vi "Match String.vi"(8 "Offset (0)":i32, 9 "Pattern":string, 11 "Source":string) -> (2 "Match?":bool, 3 "String Match":T1)   [LabVIEW 2016, in "Suggestion Box.lvclass"]
doc: "Searches in <b>Source</b> for <b>Pattern</b> starting at <b>Offset</b>.\n--------------------\nCopyright (c) 2019 Analog Devices, Inc. All rights reserved.\n\nRedistribution and use in source and binary forms, with or without modification,\nare permitted provided that the following conditions are met:\n - Redistributions of source code must retain the above copyright notice, this\n list of conditions and the following disclaimer.\n - Redistributions in binary form must reproduce the above copyright notice,\n this list of conditions and the following disclaimer in the documentation\n and/or other materials provided with the distribution.\n - Modified versions of the software must be conspicuously marked as such.\n - This software is licensed solely and exclusively for use with\n processors/products manufactured by or for Analog Devices, Inc.\n - This software may not be combined or merged with other code in any manner\n that would cause the software to become subject to terms and conditions\n which differ from those listed here.\n - Neither the name of Analog Devices, Inc. nor the names of its contributors\n may be used to endorse or promote products derived from this software\n without specific prior written permission.\n - The use of this software may or may not infringe the patent rights of one or\n more patent holders. This license does not release you from the requirement\n that you obtain separate licenses from these patent holders to use this\n software.\n\nTHIS SOFTWARE IS PROVIDED BY ANALOG DEVICES, INC. AND CONTRIBUTORS \"AS IS\" AND\nANY EXPRESS OR IMPLIED WARRANTIES, INCLUDING, BUT NOT LIMITED TO,\nNON-INFRINGEMENT, TITLE, MERCHANTABILITY AND FITNESS FOR A PARTICULAR PURPOSE\nARE DISCLAIMED. IN NO EVENT SHALL ANALOG DEVICES, INC. OR CONTRIBUTORS BE LIABLE\nFOR ANY DIRECT, INDIRECT, INCIDENTAL, SPECIAL, EXEMPLARY, PUNITIVE OR\nCONSEQUENTIAL DAMAGES (INCLUDING, BUT NOT LIMITED TO, DAMAGES ARISING OUT OF\nCLAIMS OF INTELLECTUAL PROPERTY RIGHTS INFRINGEMENT; PROCUREMENT OF SUBSTITUTE\nGOODS OR SERVICES; LOSS OF USE, DATA, OR PROFITS; OR BUSINESS INTERRUPTION)\nHOWEVER CAUSED AND ON ANY THEORY OF LIABILITY, WHETHER IN CONTRACT, STRICT\nLIABILITY, OR TORT (INCLUDING NEGLIGENCE OR OTHERWISE) ARISING IN ANY WAY OUT OF\nTHE USE OF THIS SOFTWARE, EVEN IF ADVISED OF THE POSSIBILITY OF SUCH DAMAGE.\n\n2019-01-10-7CBSD SLA"
uses:
  Suggestion Box.lvclass
  String Match.ctl
  Segment.ctl
panel:
  # "Copyright (c) 2019 Analog Devices, Inc.  All rights reserved.\n\nRedistribution and use in source and binary forms, with or without modification,\nare permitted provided that the following conditions are met:\n  - Redistributions of source code must retain the above copyright notice, this\n    list of conditions and the following disclaimer.\n  - Redistributions in binary form must reproduce the above copyright notice,\n    this list of conditions and the following disclaimer in the documentation\n    and/or other materials provided with the distribution.\n  - Modified versions of the software must be conspicuously marked as such.\n  - This software is licensed solely and exclusively for use with\n    processors/products manufactured by or for Analog Devices, Inc.\n  - This software may not be combined or merged with other code in any manner\n    that would cause the software to become subject to terms and conditions\n    which differ from those listed here.\n  - Neither the name of Analog Devices, Inc. nor the names of its contributors\n    may be used to endorse or promote products derived from this software\n    without specific prior written permission.\n  - The use of this software may or may not infringe the patent rights of one or\n    more patent holders.  This license does not release you from the requirement\n    that you obtain separate licenses from these patent holders to use this\n    software.\n\nTHIS SOFTWARE IS PROVIDED BY ANALOG DEVICES, INC. AND CONTRIBUTORS \"AS IS\" AND\nANY EXPRESS OR IMPLIED WARRANTIES, INCLUDING, BUT NOT LIMITED TO,\nNON-INFRINGEMENT, TITLE, MERCHANTABILITY AND FITNESS FOR A PARTICULAR PURPOSE\nARE DISCLAIMED. IN NO EVENT SHALL ANALOG DEVICES, INC. OR CONTRIBUTORS BE LIABLE\nFOR ANY DIRECT, INDIRECT, INCIDENTAL, SPECIAL, EXEMPLARY, PUNITIVE OR\nCONSEQUENTIAL DAMAGES (INCLUDING, BUT NOT LIMITED TO, DAMAGES ARISING OUT OF\nCLAIMS OF INTELLECTUAL PROPERTY RIGHTS INFRINGEMENT; PROCUREMENT OF SUBSTITUTE\nGOODS OR SERVICES; LOSS OF USE, DATA, OR PROFITS; OR BUSINESS INTERRUPTION)\nHOWEVER CAUSED AND ON ANY THEORY OF LIABILITY, WHETHER IN CONTRACT, STRICT\nLIABILITY, OR TORT (INCLUDING NEGLIGENCE OR OTHERWISE) ARISING IN ANY WAY OUT OF\nTHE USE OF THIS SOFTWARE, EVEN IF ADVISED OF THE POSSIBILITY OF SUCH DAMAGE.\n\n2019-01-10-7CBSD SLA"
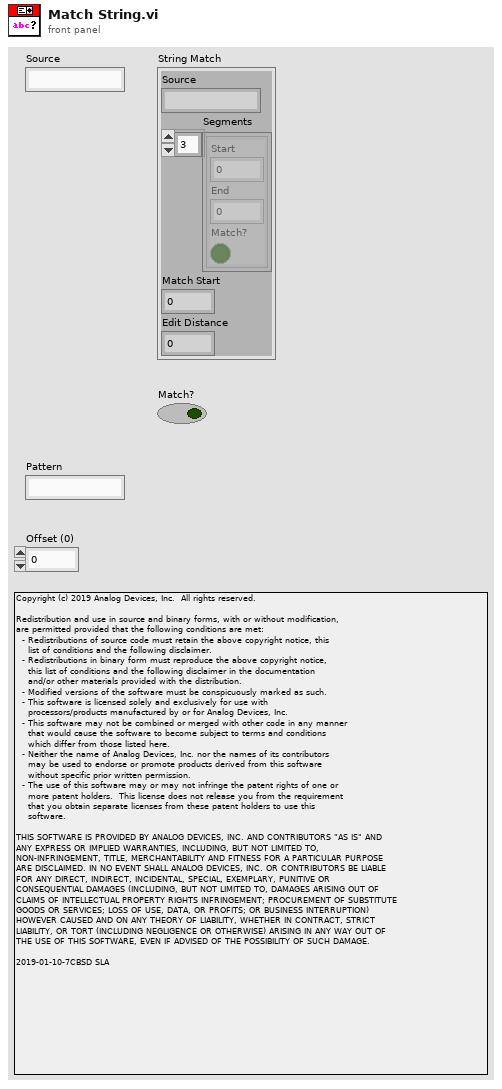
[diagram p1: front panel]
types:
  T1 = typedef "Suggestion Box.lvclass/String Match.ctl" = cluster{"Source":string, "Segments":T2[], "Match Start":i32, "Edit Distance":i32}
  T2 = typedef "Suggestion Box.lvclass/Segment.ctl" = cluster{"Start":i32, "End":i32, "Match?":bool}
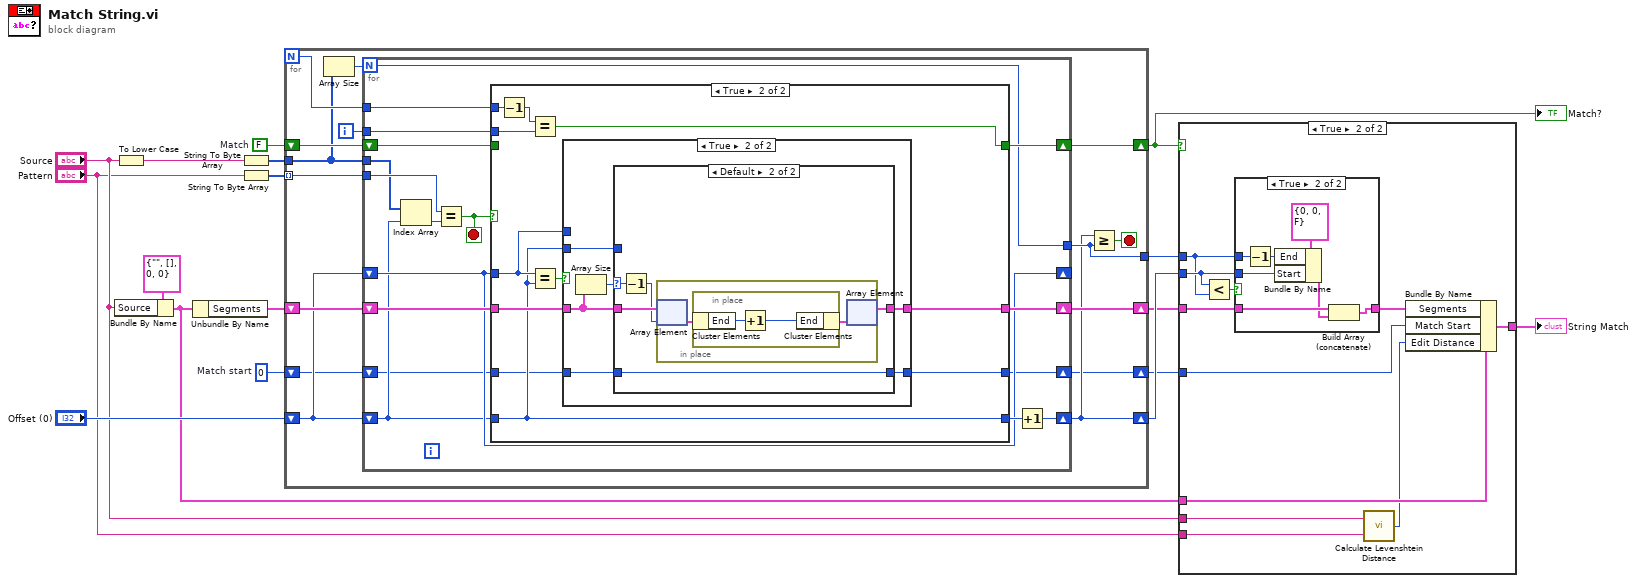
[diagram p0: block diagram]
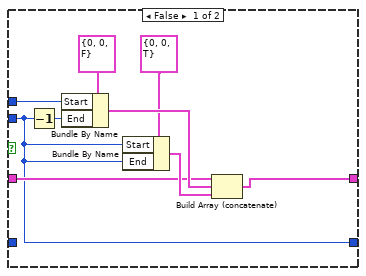
[diagram p5: hidden frame]
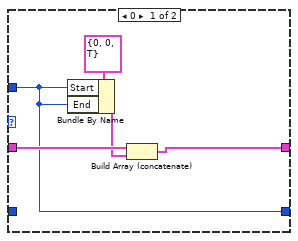
[diagram p6: hidden frame]
diagram:
  w3 = 0  # Match start
  w9 = FALSE  # Match
  n1 = Bundle By Name(cluster=T1 {"Source"="", "Segments"=[], "Match Start"=0, "Edit Distance"=0}, "Source"="Source") -> (w10:T1)
  n2 = To Lower Case(string="Source") -> (all lower case string=w16:string)
  n3 = Unbundle By Name(w10) -> ("Segments"=w8:T2[])
  n4 = String To Byte Array(string=w16) -> (unsigned byte array=w6:u8[])
  n5 = String To Byte Array(string="Pattern") -> (unsigned byte array=w5:u8[])
  n6 = for {
    N -> [w30]
    tunnel: w5 -> [w32] mode=indexing
    tunnel: w6 -> [w21]
    shift-right: [w27] -> w11
    shift-left: w8 -> [w28]
    shift-right: [w29] -> w17
    shift-left: w9 -> [w26]
    tunnel: [w24] -> w12
    shift-right: [w23] -> w15
    shift-left: "Offset (0)" -> [w22]
    shift-right: [w19] -> w4
    shift-left: w3 -> [w18]
    i -> [w31]
    stop <- w25 stop-if-true
    n7 = Array Size(array=w21) -> (size(s)=w20:i32)
    n8 = for {
      N: w20 -> [w41]
      tunnel: w21 -> [w38]
      tunnel: w32 -> [w49]
      shift-right: [w37] -> _
      shift-left: w22 -> [w37]
      tunnel: w31 -> [w48]
      tunnel: w30 -> [w47]
      shift-right: [w44] -> w27
      shift-left: w28 -> [w45]
      shift-right: [w42] -> w29
      shift-left: w26 -> [w43]
      tunnel: [w41] -> w24
      shift-right: [w39] -> w23
      shift-left: w22 -> [w35]
      shift-right: [w34] -> w19
      shift-left: w18 -> [w33]
      stop <- w46 stop-if-true
      n9 = Index Array(array=w38, index=w35) -> (element=w36:u8)
      n10 = Equal?(x=w49, y=w36) -> (x = y?=w46:bool)
      n11 = case shown="True" w46 {
        tunnel: w48 -> [_ w63]
        tunnel: w47 -> [_ w64]
        tunnel: w37 -> [_ w60]
        tunnel: w35 -> [w51 w56]
        tunnel: w45 -> [w53 w59]
        tunnel: [w53 w58] -> w44
        tunnel: w43 -> [w52 _]
        tunnel: [w52 w57] -> w42
        tunnel: [w51 w56] -> w40
        tunnel: [w50 w55] -> w34
        tunnel: w33 -> [w50 w54]
        frame False {
        }
        frame True {
          n12 = Decrement(x=w64) -> (x-1=w62:i32)
          n13 = Equal?(x=w62, y=w63) -> (x = y?=w57:bool)
          n14 = Equal?(x=w60, y=w56) -> (x = y?=w61:bool)
          n15 = case shown="True" w61 {
            tunnel: w60 -> [w73 _]
            tunnel: w56 -> [w65 w76]
            tunnel: w59 -> [w70 w78]
            tunnel: [w69 w77] -> w58
            tunnel: [w65 w75] -> w55
            tunnel: w54 -> [_ w74]
            frame False {
              n16 = Decrement(x=w65) -> (x-1=w67:i32)
              n17 = Bundle By Name(cluster=T2 {"Start"=0, "End"=0, "Match?"=FALSE} ("Array"), "Start"=w73, "End"=w67) -> (w71:T2)
              n18 = Bundle By Name(cluster=T2 {"Start"=0, "End"=0, "Match?"=TRUE} ("Array"), "Start"=w65, "End"=w65) -> (w72:T2)
              n19 = Build Array (concatenate)(w70, w71, w72) -> (w69:T2[])
            }
            frame True {
              n20 = Array Size(array=w78) -> (size(s)=w79:i32)
              n21 = case shown="Default" w79 {
                selector: w79 -> [_ w88]
                tunnel: w76 -> [w80 _]
                tunnel: w78 -> [w83 w89]
                tunnel: [w81 w86] -> w77
                tunnel: [w80 w85] -> w75
                tunnel: w74 -> [_ w85]
                frame 0 {
                  n22 = Bundle By Name(cluster=T2 {"Start"=0, "End"=0, "Match?"=TRUE} ("Array"), "Start"=w80, "End"=w80) -> (w82:T2)
                  n23 = Build Array (concatenate)(w83, w82) -> (w81:T2[])
                }
                frame Default {
                  n24 = Decrement(x=w88) -> (x-1=w87:i32)
                  n25 = in-place {
                    n26 = in-place-array #1(w89, w87) -> (w91:T2)
                    n27 = in-place {
                      n28 = in-place-cluster #2(w91) -> ("End"=w93:i32)
                      n29 = Increment(x=w93) -> (x+1=w92:i32)
                      n30 = in-place-cluster #2("End"=w92) -> (w90:T2)
                    }
                    n31 = in-place-array #1(w90) -> (w86:T2[])  [unwired: 1 out]
                  }
                }
              }
            }
          }
        }
      }
      n32 = Increment(x=w40) -> (x+1=w39:i32)
    }
    n33 = Greater Or Equal?(x=w23, y=w24) -> (x >= y?=w25:bool)
  }
  "Match?" <- w17
  n34 = case shown="True" w17 {
    tunnel: w10 -> [_ w104]
    tunnel: w11 -> [_ w103]
    tunnel: [_ w98] -> w13
    tunnel: w15 -> [_ w101]
    tunnel: w12 -> [_ w100]
    tunnel: w4 -> [_ w97]
    tunnel: "Source" -> [_ w96]
    tunnel: "Pattern" -> [_ w95]
    frame False {
    }
    frame True {
      n35 = Less?(x=w101, y=w100) -> (x < y?=w99:bool)
      n36 = case shown="True" w99 {
        tunnel: w103 -> [w105 w112]
        tunnel: [w105 w111] -> w102
        tunnel: w101 -> [_ w110]
        tunnel: w100 -> [_ w109]
        frame False {
        }
        frame True {
          n37 = Decrement(x=w109) -> (x-1=w106:i32)
          n38 = Bundle By Name(cluster=T2 {"Start"=0, "End"=0, "Match?"=FALSE} ("Array"), "End"=w106, "Start"=w110) -> (w107:T2)
          n39 = Build Array (concatenate)(w112, w107) -> (w111:T2[])
        }
      }
      n40 = call "Calculate Levenshtein Distance.vi"("Pattern"=w95, "Source"=w96) -> ("Distance"=w94:i32)
      n41 = Bundle By Name(cluster=w104, "Segments"=w102, "Match Start"=w97, "Edit Distance"=w94) -> (w98:T1)
    }
  }
  "String Match" <- w13
